vi "Adapt to inputs.vi"(3 "Term Types":T1, 4 "XRef":refnum<vi>, 5 "State In":T5) -> (0 "Reply":string[](array[string]), 2 "State Out":T5)   [LabVIEW 2012, in "ArrayDimension.xnode"]
uses:
  ArrayDimension.xnode
  State.ctl
  <vilib>/XNodeSupport/XNodeTermTypeIDPairs.ctl
  <vilib>/XNodeSupport/XNodeTermTypeIDPair.ctl
  <vilib>/XNodeSupport/XNodeType.ctl
  <vilib>/XNodeSupport/XNodeString.ctl
  <vilib>/Utility/VariantDataType/VariantType.lvlib
  <vilib>/XNodeSupport/NI_XNodeSupport.lvlib
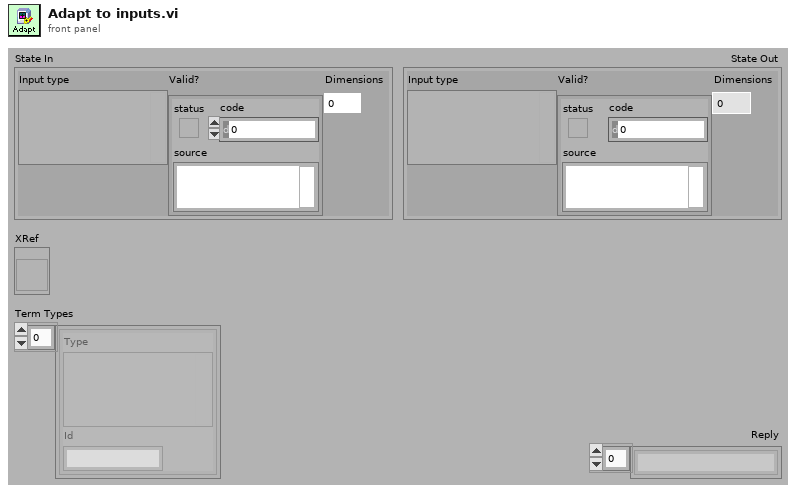
[diagram p1: front panel]
types:
  T1 = typedef "NI_XNodeSupport.lvlib/XNodeTermTypeIDPairs.ctl" = T2[]
  T2 = typedef "NI_XNodeSupport.lvlib/XNodeTermTypeIDPair.ctl" = cluster{"Type":T3, "Id":T4}
  T3 = typedef "NI_XNodeSupport.lvlib/XNodeType.ctl" = variant
  T4 = typedef "NI_XNodeSupport.lvlib/XNodeString.ctl" = string
  T5 = typedef "ArrayDimension.xnode/State.ctl" = cluster{"Input type":variant, "Valid?":errorcluster, "Dimensions":i32}
  T6 = typedef "VariantType.lvlib/Type.ctl" = enum8{"Invalid Type", "Void", "I8", "I16", "I32", "I64", "U8", "U16", "U32", "U64", "Single Float", "Double Float", "Extended Float", "Single Complex", "Double Complex", "Extended Complex", "Enum U8", "Enum U16", "Enum U32", "Enum U64", "Single Float With Unit", "Double Float With Unit", "Extended Float With Unit", "Single Complex with Unit", "Double Complex with Unit", "Extended Complex with Unit", "Boolean", "String", "Path", "Picture", "Tag", "Array", "Cluster", "Variant", "LV Variant", "Waveform", "Timestamp", "Digital Waveform", "Digital Data", "ExpressData", "Refnum", "External Data", "VI", "Poly VI", "LabVIEW Class Instance", "Fixed Point"}
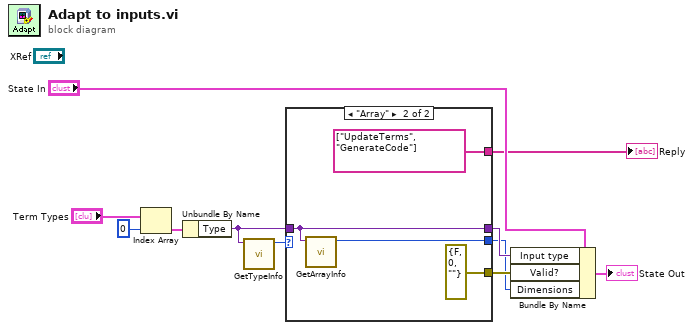
[diagram p0: block diagram]
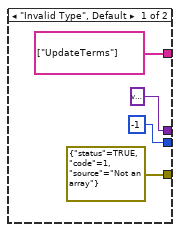
[diagram p2: hidden frame]
diagram:
  n1 = Index Array(array="Term Types", index=0) -> (element=w9:T2)
  n2 = Unbundle By Name(w9) -> ("Type"=w3:T3)
  n3 = call <vilib>:"GetTypeInfo.vi"("Variant"=w3) -> ("Type Enum"=w2:T6)  [unwired: 1 in, 9 out]
  n4 = case shown="\"Array\"" w2 {
    tunnel: w3 -> [_ w17]
    tunnel: [variant ("Input type") w17] -> w6
    tunnel: [errorcluster {"status"=TRUE, "code"=1, "source"="Not an array"} ("Valid?") errorcluster {"status"=FALSE, "code"=0, "source"=""} ("Valid?")] -> w5
    tunnel: [string[] ["UpdateTerms"] string[] ["UpdateTerms", "GenerateCode"] ("Reply")] -> w4
    tunnel: [-1 ("NDims") w16] -> w1
    frame "Invalid Type", Default {
    }
    frame "Array" {
      n5 = call <vilib>:"GetArrayInfo.vi"("Variant"=w17) -> ("NDims"=w16:i32)  [unwired: 1 in, 9 out]
    }
  }
  "Reply" <- w4
  n6 = Bundle By Name(cluster="State In", "Input type"=w6, "Valid?"=w5, "Dimensions"=w1) -> (→"State Out":T5)
